vi "EndTestSuiteCalled.vi"(1 "FakeTestListener In":refnum<class "FakeTestListener.lvclass">) -> (0 "EndTestSuite Called":bool)   [LabVIEW 2019, in "TestResultTest.lvlib" / "Support.lvlib" / "FakeTestListener.lvclass"]
uses:
  FakeTestListener.lvclass
  FakeTestListener.lvclass/FakeTestListener.ctl
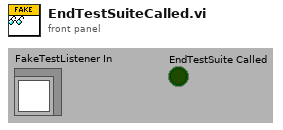
[diagram p1: front panel]
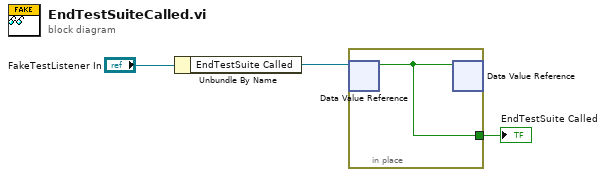
[diagram p0: block diagram]
diagram:
  n1 = Unbundle By Name("FakeTestListener In") -> ("EndTestSuite Called"=w3:refnum<data-value>)
  n2 = in-place {
    in-place-border: [w4] -> w2
    n3 = in-place-dvr #1(w3) -> (w4:bool)  [unwired: 1 out]
    n4 = in-place-dvr #1(w4) -> ()  [unwired: 2 out]
  }
  "EndTestSuite Called" <- w2
